vi "Tarf Angle Updater.vi"() -> ()   [LabVIEW 2012]
uses:
  Robot Global Data.vi
panel:
  out "Distance 2":dbl
  out "Angle Right":dbl
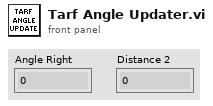
[diagram p1: front panel]
types:
  T1 = typedef "WPI_EncoderDevRef.ctl" = cluster{"DevStatus":errorcluster, "EncoderIndex":T2, "CounterIndex":T3, "DistancePerCount":dbl, "Decoding Type":T4}
  T2 = typedef "FPGA_EncoderIdx.ctl" = enum8{"Enc 0", "Enc 1", "Enc 2", "Enc 3", "Invalid"}
  T3 = typedef "FPGA_CounterCtrSystemIndex.ctl" = enum8{"Ctr 0", "Ctr 1", "Ctr 2", "Ctr 3", "Ctr 4", "Ctr 5", "Ctr 6", "Ctr 7", "Invalid"}
  T4 = typedef "WPI_EncoderType.ctl" = enum16{"1x", "2x", "4x"}
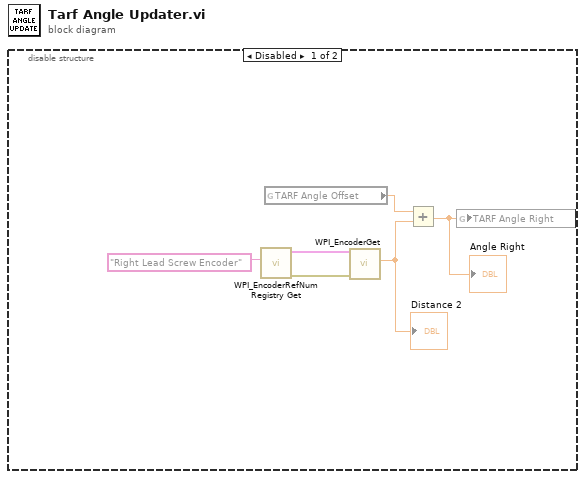
[diagram p0: block diagram]
diagram:
  n1 = disable-structure shown="Disabled" {
    frame Disabled {
      n2 = call <vilib>:"WPI_EncoderRefNum Registry Get.vi"("refnum name"="Right Lead Screw Encoder") -> ("error out"=w4:errorcluster, "EncoderDevRef"=w5:T1)  [unwired: 9 in]
      n3 = global read "Robot Global Data.vi" "TARF Angle Offset"() -> (w3:dbl)
      n4 = call <vilib>:"WPI_EncoderGet.vi"("error in (no error)"=w4, "EncoderDevRef"=w5) -> ("Distance"=w2:dbl)  [unwired: 4 in, 5 out]
      "Distance 2" <- w2
      n5 = Add(x=w3, y=w2) -> (x+y=w1:dbl)
      "Angle Right" <- w1
      n6 = global write "Robot Global Data.vi" "TARF Angle Right"(w1) -> ()
    }
    frame Enabled {
    }
  }
